vi "Waveform Generation User Interface.vi"() -> ()   [LabVIEW 2023, in "GUI.lvlib" / "Diagnostic.lvlib"]
uses:
  Diagnostic.lvlib
  Control/Waveform Generation 6739.ctl
  Control/Waveform Generation.ctl
  Control/Waveform Generation 6738.ctl
  HardwareAbstractionLayer_LVOOP/Analog Output/NI Waveform Output_class/NI Waveform Output.lvclass
  D:/eDCU LTT/VT LTT Project/Source Code/HardwareAbstractionLayer_LVOOP/Analog Output/AO/AO.lvclass
  HardwareAbstractionLayer_LVOOP/Database/SQL Public VI/Control/DB Options.ctl
  HardwareAbstractionLayer_LVOOP/Main/Class Ref.ctl
  HardwareAbstractionLayer_LVOOP/DMM/DMM.lvclass
  HardwareAbstractionLayer_LVOOP/Function Generator/Function Generator.lvclass
  HardwareAbstractionLayer_LVOOP/Oscilloscope/Oscilloscope.lvclass
  HardwareAbstractionLayer_LVOOP/PowerSupply/PowerSupply.lvclass
  HardwareAbstractionLayer_LVOOP/Teststand/Teststand.lvclass
  HardwareAbstractionLayer_LVOOP/Analog Output/AO/AO.lvclass
  HardwareAbstractionLayer_LVOOP/Analog Input/AI/AI.lvclass
  HardwareAbstractionLayer_LVOOP/Database/Database.lvclass
  HardwareAbstractionLayer_LVOOP/Digital Output/DO_class/DO.lvclass
  HardwareAbstractionLayer_LVOOP/Digital Input/DI_class/DI.lvclass
  HardwareAbstractionLayer_LVOOP/PWM Output/PWM Output_class/PWM Output.lvclass
  HardwareAbstractionLayer_LVOOP/PWM Input/PWM Input_class/PWM Input.lvclass
  HardwareAbstractionLayer_LVOOP/NI Switch/NISwitch_class/NISwitch.lvclass
  HardwareAbstractionLayer_LVOOP/Modbus/Modbus_class/Modbus.lvclass
  HardwareAbstractionLayer_LVOOP/CAN/CAN Lib/CAN_class/CAN.lvclass
  HardwareAbstractionLayer_LVOOP/Main/Main.lvclass
panel:
  in  "Stop Acquire":bool
  in  "Start Acquire":bool
  out "error out":errorcluster
  in  "error in":errorcluster
  in  "Operation":T1(tab)
  in  "PXIe - 6739 M1":T2
  in  "PXIe - 6739 M2":T2
  in  "PXIe - 6738 M1":T4
  in  "Stop":bool caption="Blank"
  # "Analog Waveform Generation"
  # "Operation:"
  # "Waveform Type"
  # "Frequency"
  # "Amplitude"
  # "Phase"
  # "Waveform Type"
  # "Frequency"
  # "Amplitude"
  # "Phase"
  # "Waveform Type"
  # "Frequency"
  # "Amplitude"
  # "Phase"
  # "Waveform Type"
  # "Frequency"
  # "Amplitude"
  # "Phase"
  # "Waveform Type"
  # "Frequency"
  # "Amplitude"
  # "Phase"
  # "Waveform Type"
  # "Frequency"
  # "Amplitude"
  # "Phase"
  # "Waveform Type"
  # "Frequency"
  # "Amplitude"
  # "Phase"
  # "Waveform Type"
  # "Frequency"
  # "Amplitude"
  # "Phase"
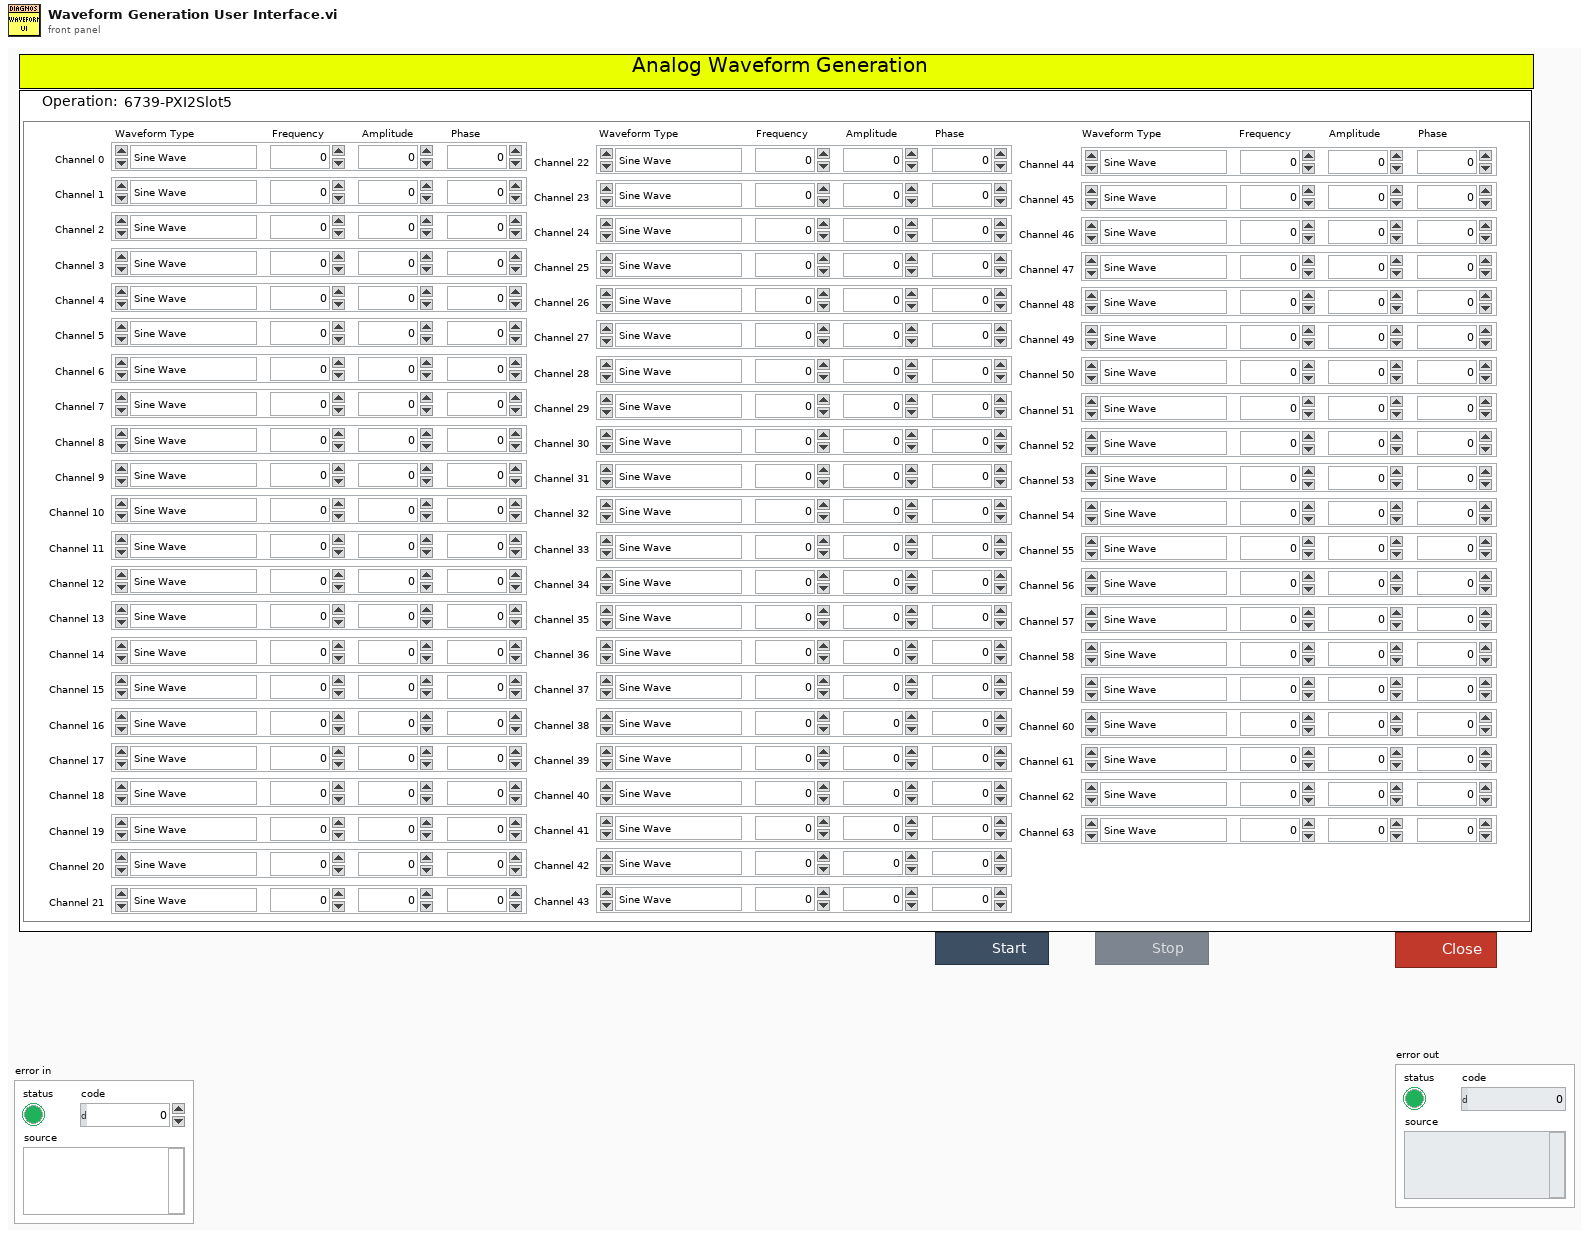
[diagram p1: front panel]
types:
  T1 = enum32{"6739-PXI2Slot5", "6739-PXI2Slot6", "6738-PXI2Slot4"}
  T2 = typedef "GUI.lvlib/Diagnostic.lvlib/Waveform Generation 6739.ctl" = cluster{"Channel 0":T3, "Channel 1":T3, "Channel 2":T3, "Channel 3":T3, "Channel 4":T3, "Channel 5":T3, "Channel 6":T3, "Channel 7":T3, "Channel 8":T3, "Channel 9":T3, "Channel 10":T3, "Channel 11":T3, "Channel 12":T3, "Channel 13":T3, "Channel 14":T3, "Channel 15":T3, "Channel 16":T3, "Channel 17":T3, "Channel 18":T3, "Channel 19":T3, "Channel 20":T3, "Channel 21":T3, "Channel 22":T3, "Channel 23":T3, "Channel 24":T3, "Channel 25":T3, "Channel 26":T3, "Channel 27":T3, "Channel 28":T3, "Channel 29":T3, "Channel 30":T3, "Channel 31":T3, "Channel 32":T3, "Channel 33":T3, "Channel 34":T3, "Channel 35":T3, "Channel 36":T3, "Channel 37":T3, "Channel 38":T3, "Channel 39":T3, "Channel 40":T3, "Channel 41":T3, "Channel 42":T3, "Channel 43":T3, "Channel 44":T3, "Channel 45":T3, "Channel 46":T3, "Channel 47":T3, "Channel 48":T3, "Channel 49":T3, "Channel 50":T3, "Channel 51":T3, "Channel 52":T3, "Channel 53":T3, "Channel 54":T3, "Channel 55":T3, "Channel 56":T3, "Channel 57":T3, "Channel 58":T3, "Channel 59":T3, "Channel 60":T3, "Channel 61":T3, "Channel 62":T3, "Channel 63":T3}
  T3 = typedef "GUI.lvlib/Diagnostic.lvlib/Waveform Generation.ctl" = cluster{"Waveform Type":enum16{"Sine Wave", "Triangle Wave", "Square Wave", "Sawtooth Wave"}, "Amplitude":dbl, "Frequency":dbl, "Phase":dbl}
  T4 = typedef "GUI.lvlib/Diagnostic.lvlib/Waveform Generation 6738.ctl" = cluster{"Channel 0":T3, "Channel 1":T3, "Channel 2":T3, "Channel 3":T3, "Channel 4":T3, "Channel 5":T3, "Channel 6":T3, "Channel 7":T3, "Channel 8":T3, "Channel 9":T3, "Channel 10":T3, "Channel 11":T3, "Channel 12":T3, "Channel 13":T3, "Channel 14":T3, "Channel 15":T3, "Channel 16":T3, "Channel 17":T3, "Channel 18":T3, "Channel 19":T3, "Channel 20":T3, "Channel 21":T3, "Channel 22":T3, "Channel 23":T3, "Channel 24":T3, "Channel 25":T3, "Channel 26":T3, "Channel 27":T3, "Channel 28":T3, "Channel 29":T3, "Channel 30":T3, "Channel 31":T3}
  T5 = typedef "HardwareAbstractionLayer_LVOOP.lvlib/Database.lvclass/DB Options.ctl" = enum16{"Init", "Select Data", "Insert Data", "Update Data", "Delete Data", "Execute Query", "Create Schema", "Create Table", "List Tables", "List Columns", "Close"}
  T6 = typedef "HardwareAbstractionLayer_LVOOP.lvlib/Main.lvclass/Class Ref.ctl" = cluster{"DMM":refnum<class "DMM.lvclass">, "Function Generator":refnum<class "Function Generator.lvclass">, "Oscilloscope":refnum<class "Oscilloscope.lvclass">, "PowerSupply":refnum<class "PowerSupply.lvclass">, "Teststand":refnum<class "Teststand.lvclass">, "AO":refnum<class "AO.lvclass">, "AI":refnum<class "AI.lvclass">, "Database":refnum<class "Database.lvclass">, "AO Waveform Generation":refnum<class "AO.lvclass">, "DO":refnum<class "DO.lvclass">, "DI":refnum<class "DI.lvclass">, "PWM Output":refnum<class "PWM Output.lvclass">, "PWM Input":refnum<class "PWM Input.lvclass">, "RelayOutput":refnum<class "NISwitch.lvclass">, "Modbus":refnum<class "Modbus.lvclass">, "CAN":refnum<class "CAN.lvclass">}
  T7 = enum8{"Enabled", "Disabled", "Disabled and Grayed Out"}
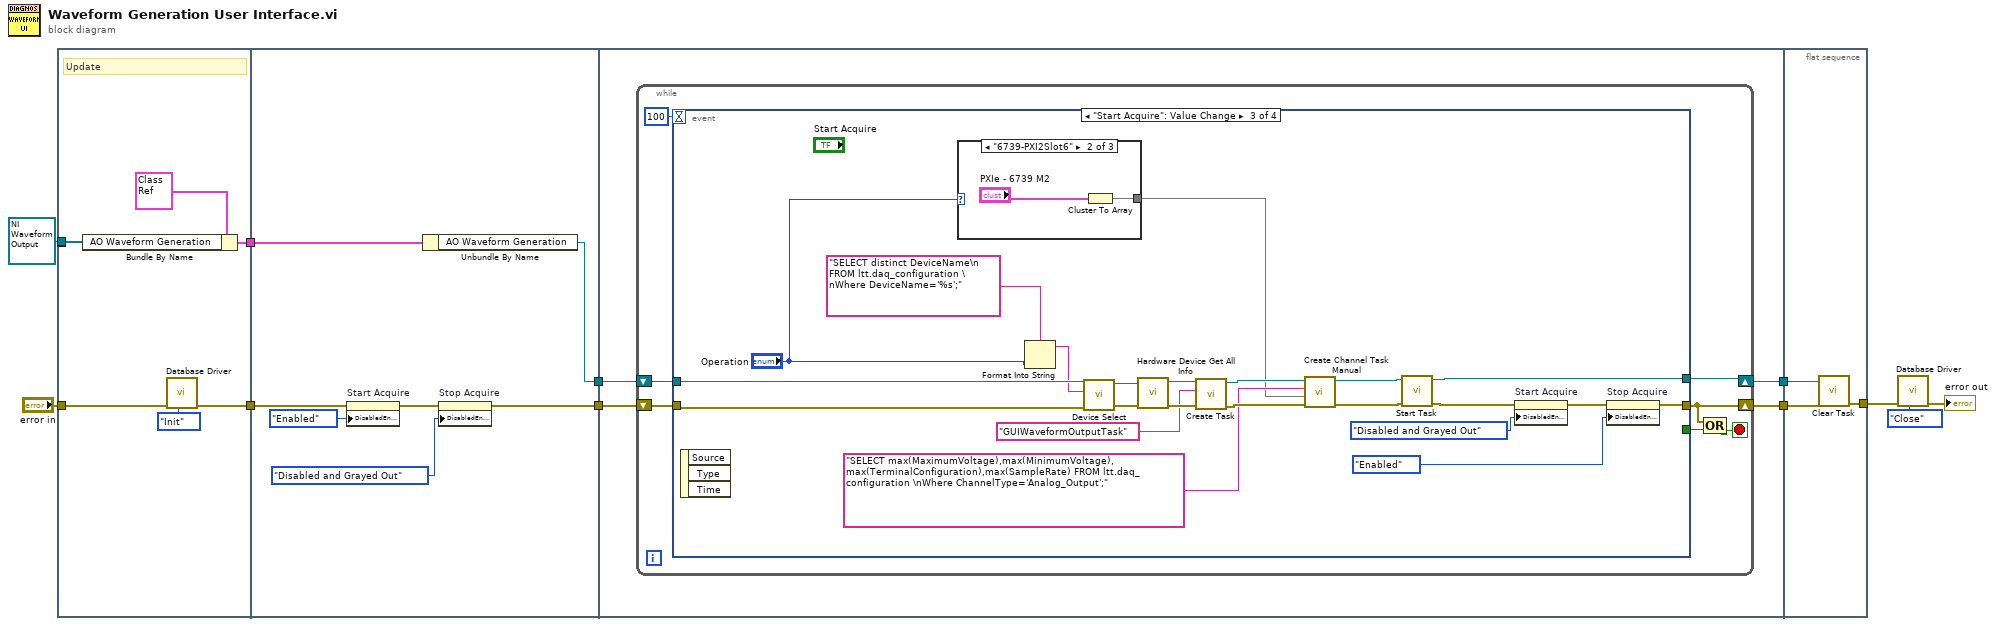
[diagram p0: block diagram]
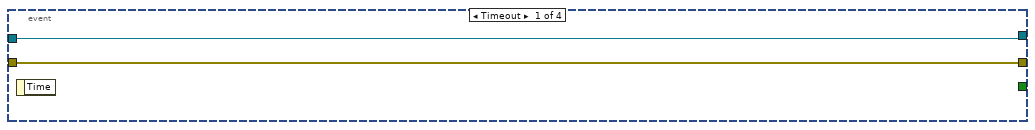
[diagram p2: hidden frame]
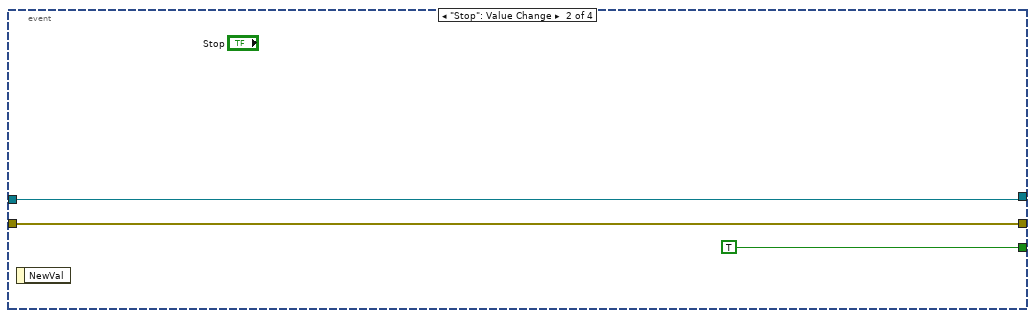
[diagram p3: hidden frame]
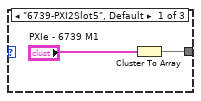
[diagram p4: hidden frame]
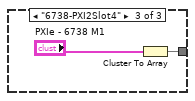
[diagram p5: hidden frame]
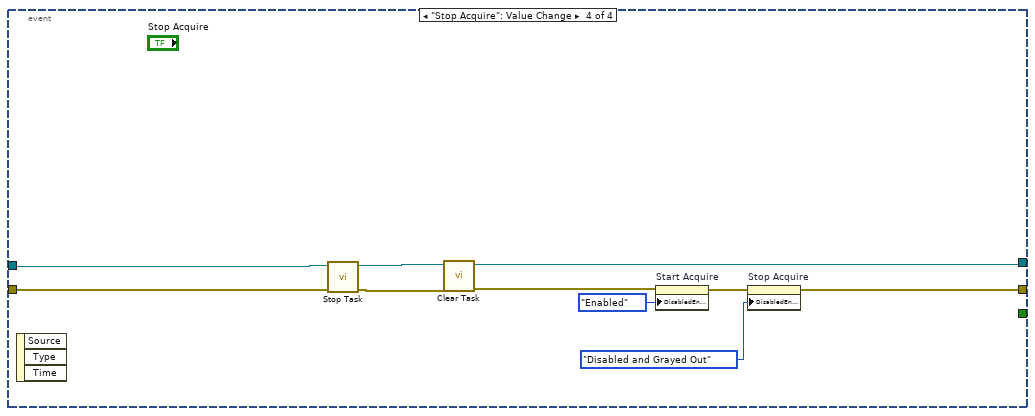
[diagram p6: hidden frame]
diagram:
  n1 = flat-sequence {
    tunnel: "error in" -> [w17]
    tunnel: [w13] -> w10
    tunnel: [w14] -> _
    tunnel: [w15] -> w8
    tunnel: refnum<class "NI Waveform Output.lvclass"> refnum ("HardwareAbstractionLayer_LVOOP.lvlib:NI Waveform Output.lvclass") -> [w14]
    tunnel: w10 -> [w22]
    tunnel: [w18] -> w9
    tunnel: w8 -> [w24]
    tunnel: [w23] -> w7
    tunnel: w9 -> [w28]
    tunnel: w7 -> [w27]
    tunnel: [w26] -> w4
    tunnel: [w25] -> w3
    tunnel: [w79] -> w6
    tunnel: w4 -> [w81]
    tunnel: w3 -> [w80]
    frame #0 {
      # "Update"
      n2 = Bundle By Name(cluster=T6 {"DMM"=refnum, "Function Generator"=refnum, "Oscilloscope"=refnum, "PowerSupply"=refnum, "Teststand"=refnum, "AO"=refnum, "AI"=refnum, "Database"=refnum, "AO Waveform Generation"=refnum, "DO"=refnum, "DI"=refnum, "PWM Output"=refnum, "PWM Input"=refnum, "RelayOutput"=refnum, "Modbus"=refnum, "CAN"=refnum} ("Class Cluster"), "AO Waveform Generation"=w14) -> (w15:T6)
      n3 = call "Database Driver.vi"("Options"=DB_Options."Init", "error in"=w17) -> ("error out"=w13:errorcluster)  [unwired: 6 in, 3 out]
    }
    frame #1 {
      n4 = property on="Start Acquire" class="Bool"(error in=w22, "DisabledEnum"=T7."Enabled" ("Disabled")) -> (error out=w21:errorcluster)  [unwired: 1 in, 1 out]
      n5 = Unbundle By Name(w24) -> ("AO Waveform Generation"=w23:refnum<class "AO.lvclass">)
      n6 = property on="Stop Acquire" class="Bool"(error in=w21, "DisabledEnum"=T7."Disabled and Grayed Out" ("Disabled")) -> (error out=w18:errorcluster)  [unwired: 1 in, 1 out]
    }
    frame #2 {
      n7 = while {
        shift-right: [w29] -> w26
        shift-left: w28 -> [w33]
        shift-right: [w32] -> w25
        shift-left: w27 -> [w34]
        stop <- w30 stop-if-true
        n8 = event shown="[2] \"Start Acquire\": Value Change" {
          selector: _ -> [_ _ _ _]
          dyn-events: _ -> [_ _ _ _]
          timeout: 100 -> [_ _ _ _]
          tunnel: [_ TRUE ("Stop") _ _] -> w31
          tunnel: w34 -> [w37 w39 w56 w73]
          tunnel: w33 -> [w36 w38 w57 w72]
          tunnel: [w37 w39 w46 w78] -> w32
          tunnel: [w36 w38 w48 w69] -> w29
          event Timeout {
            n9 = event-data() -> ()  [unwired: 1 in, 1 out]
          }
          event "Stop": Value Change {
            n10 = event-data() -> ()  [unwired: 1 in, 1 out]
          }
          event "Start Acquire": Value Change {
            n11 = event-data() -> ()  [unwired: 1 in, 3 out]
            n12 = case shown="\"6739-PXI2Slot6\"" "Operation" {
              tunnel: [w63 w65 w67] -> w49
              frame "6739-PXI2Slot5", Default {
                n13 = Cluster To Array(cluster="PXIe - 6739 M1") -> (array=w63:T3[])
              }
              frame "6739-PXI2Slot6" {
                n14 = Cluster To Array(cluster="PXIe - 6739 M2") -> (array=w65:T3[])
              }
              frame "6738-PXI2Slot4" {
                n15 = Cluster To Array(cluster="PXIe - 6738 M1") -> (array=w67:T3[])
              }
            }
            n16 = Format Into String(format string="SELECT distinct DeviceName\n FROM ltt.daq_configuration \nWhere DeviceName='%s';" ("SQL query"), "Operation") -> (resulting string=w41:string)  [unwired: 2 in, 1 out]
            n17 = call-dynamic "Device Select.vi"("error in (no error)"=w57, "SQL query"=w41, "AO in"=w56) -> ("error out"=w61:errorcluster, "AO out"=w62:refnum<class "AO.lvclass">)  [unwired: 7 in]
            n18 = call-dynamic "Hardware Device Get All Info.vi"("error in (no error)"=w61, "AO in"=w62) -> ("error out"=w59:errorcluster, "AO out"=w60:refnum<class "AO.lvclass">)  [unwired: 8 in]
            n19 = call-dynamic "Create Task.vi"("error in (no error)"=w59, "Task name"="GUIWaveformOutputTask", "AO in"=w60) -> ("error out"=w51:errorcluster, "AO out"=w52:refnum<class "AO.lvclass">)  [unwired: 7 in]
            n20 = call-dynamic "Create Channel Task Manual.vi"("error in (no error)"=w51, "Waveform Generation"=w49, "SQL query"="SELECT max(MaximumVoltage),max(MinimumVoltage), max(TerminalConfiguration),max(SampleRate) FROM ltt.daq_configuration \nWhere ChannelType='Analog_Output';", "AO in"=w52) -> ("error out"=w45:errorcluster, "AO out"=w47:refnum<class "AO.lvclass">)  [unwired: 6 in]
            n21 = call-dynamic "Start Task.vi"("error in (no error)"=w45, "AO in"=w47) -> ("error out"=w44:errorcluster, "AO out"=w46:refnum<class "AO.lvclass">)  [unwired: 8 in]
            n22 = property on="Start Acquire" class="Bool"(error in=w44, "DisabledEnum"=T7."Disabled and Grayed Out" ("Disabled")) -> (error out=w53:errorcluster)  [unwired: 1 in, 1 out]
            n23 = property on="Stop Acquire" class="Bool"(error in=w53, "DisabledEnum"=T7."Enabled" ("Disabled")) -> (error out=w48:errorcluster)  [unwired: 1 in, 1 out]
          }
          event "Stop Acquire": Value Change {
            n24 = event-data() -> ()  [unwired: 1 in, 3 out]
            n25 = call-dynamic "Stop Task.vi"("error in (no error)"=w72, "AO in"=w73) -> ("error out"=w71:errorcluster, "AO out"=w70:refnum<class "AO.lvclass">)  [unwired: 8 in]
            n26 = call-dynamic "Clear Task.vi"("error in (no error)"=w71, "AO in"=w70) -> ("error out"=w74:errorcluster, "AO out"=w78:refnum<class "AO.lvclass">)  [unwired: 8 in]
            n27 = property on="Start Acquire" class="Bool"(error in=w74, "DisabledEnum"=T7."Enabled" ("Disabled")) -> (error out=w75:errorcluster)  [unwired: 1 in, 1 out]
            n28 = property on="Stop Acquire" class="Bool"(error in=w75, "DisabledEnum"=T7."Disabled and Grayed Out" ("Disabled")) -> (error out=w69:errorcluster)  [unwired: 1 in, 1 out]
          }
        }
        n29 = Compound Arithmetic op=OR(w29, w31) -> (w30:bool)
      }
    }
    frame #3 {
      n30 = call-dynamic "Clear Task.vi"("error in (no error)"=w81, "AO in"=w80) -> ("error out"=w79:errorcluster)  [unwired: 8 in, 1 out]
    }
  }
  n31 = call "Database Driver.vi"("Options"=DB_Options."Close", "error in"=w6) -> ("error out"=→"error out":errorcluster)  [unwired: 6 in, 3 out]
